vi "PDFcreator.vi"() -> ()   [LabVIEW 2015]
uses:
  <vilib>/Utility/NIReport.llb/NI_report.lvclass
  <vilib>/Utility/NIReport.llb/Append Report Text (str wrap).vi
  <vilib>/Utility/NIReport.llb/Word/NI_Word.lvclass
panel:
  in  "text options":T1
  in  "font settings":T2={"Charset (-1)"=-1, "Weight (-1)"=-1, "Name"="", "Size"=" "}
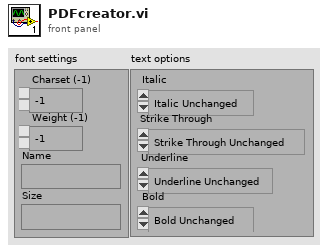
[diagram p1: front panel]
types:
  T1 = cluster{"Italic":enum16{"Italic Unchanged", "Italic On", "Italic Off"}, "Strike Through":enum16{"Strike Through Unchanged", "Strike Through On", "Strike Through Off"}, "Underline":enum16{"Underline Unchanged", "Underline On", "Underline Off"}, "Bold":enum16{"Bold Unchanged", "Bold On", "Bold Off"}}
  T2 = cluster{"Charset (-1)":i16, "Weight (-1)":i16, "Name":string, "Size":string}
  T3 = enum16{"Standard Report", "HTML", "Word", "Excel"}
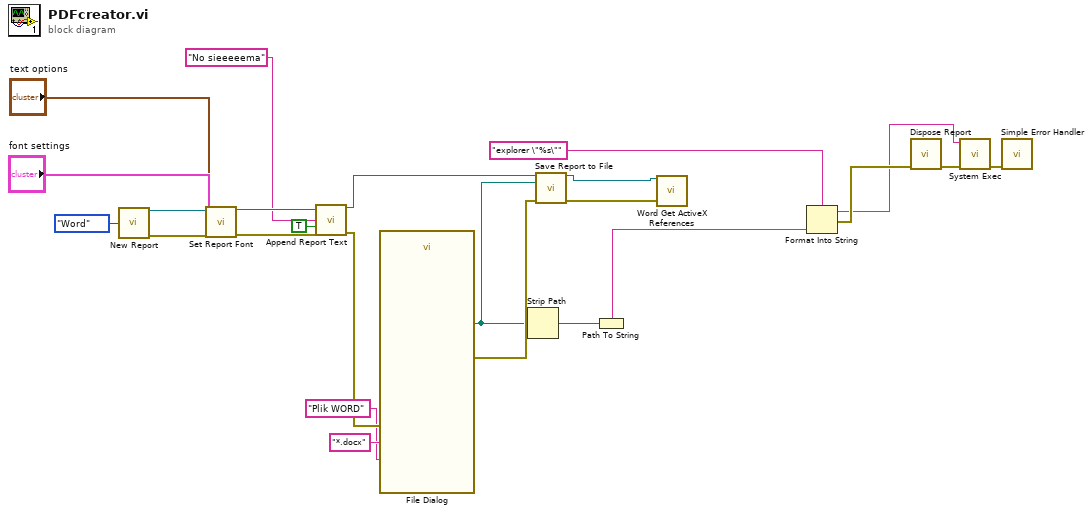
[diagram p0: block diagram]
diagram:
  n1 = call <vilib>:"New Report.vi"("report type"=T3."Word") -> ("report out"=w23:refnum<class "NI_report.lvclass">, "error out"=w20:errorcluster)  [unwired: 13 in]
  n2 = call-dynamic "Set Report Font.vi"("report in"=w23, "text options"="text options", "font settings"="font settings", "error in (no error)"=w20) -> ("report out"=w22:refnum<class "NI_report.lvclass">, "error out"=w19:errorcluster)  [unwired: 9 in, 1 out]
  n3 = call-poly <vilib>:"Append Report Text.vi"("report in"=w22, "text"="No sieeeeema", "append on new line? (F)"=TRUE, "error in (no error)"=w19) -> ("report out"=w21:refnum<class "NI_report.lvclass">, "error out"=w18:errorcluster)  [unwired: 8 in, 2 out]
  n4 = call "File Dialog"("error in"=w18, "pattern (all files)"="*.docx", "pattern label"="Plik WORD" ("default name")) -> ("selected path"=w10:path, "error out"=w17:errorcluster)  [unwired: 9 in, 2 out]
  n5 = Strip Path(path=w10) -> (stripped path=w3:path)  [unwired: 1 out]
  n6 = call-dynamic "Save Report to File.vi"("report in"=w21, "report file path"=w10, "error in (no error)"=w17) -> ("report out"=w1:refnum<class "NI_report.lvclass">, "error out"=w2:errorcluster)  [unwired: 11 in]
  n7 = Path To String(path=w3) -> (string=w6:string)
  n8 = call <vilib>:"Word Get ActiveX References.vi"("report in"=w1, "error in (no error)"=w2) -> ()  [unwired: 7 in, 7 out]
  n9 = Format Into String(format string="explorer \"%s\"", w6) -> (resulting string=w5:string, error out=w9:errorcluster)  [unwired: 2 in]
  n10 = call-dynamic "Dispose Report.vi"("error in (no error)"=w9) -> ("error out"=w8:errorcluster)  [unwired: 14 in]
  n11 = call <vilib>:"System Exec.vi"("error in (no error)"=w8, "command line"=w5) -> ("error out"=w7:errorcluster)  [unwired: 6 in, 3 out]
  n12 = call <vilib>:"Simple Error Handler.vi"("error in (no error)"=w7) -> ()  [unwired: 4 in, 5 out]
